vi "Sort 1D Array (U8)__ogtk.vi"(9 "Order":enum16{"ascending", "descending"}(ring), 11 "Array in":u8[](array[numeric])) -> (2 "Sorted Pointers":i32[](array[numeric]), 3 "Sorted Array out":u8[](array[numeric]))   [LabVIEW 2018]
doc: "This polymorphic VI sorts a 1D array of numerics or strings, regardless of the array size. You can specify whether to sort in ascending or descending order."
panel:
  # "Sort 1D Array\n\nThis VI sorts a 1D array of any size in descending or ascending order.\n\nPlease visit http://www.OpenG.org to learn about the\nOpen Source LabVIEW software movement.\n\nNOTICE -- YOU MUST LEAVE THIS NOTICE IN PLACE.  PER THE TERMS OF THE LICENSE BELOW, YOU MAY SUBLICENSE THIS SOFTWARE \nIN ANY WAY THAT DOES NOT CONFLICT WITH THIS LICENSE.\n\n### BSD License (http://www.opensource.org/licenses/bsd-license.php) Begin ###\n \nCopyright (c) 2002, Jim Kring <jim@jimkring.com>\nCopyright (c) 2002, Cal-Bay Systems, Inc. <info@calbay.com>\nCopyright (c) 2005, MKS Instruments, Inc., author: Doug Femec<doug_femec@mksinst.com>, IM dafemec\n\nAll rights reserved.\n\nRedistribution and use in source and binary forms, with or without modification, are permitted provided that the following conditions are met:\n\n    * Redistributions of source code must retain the above copyright notice, this list of conditions and the following disclaimer.\n    * Redistributions in binary form must reproduce the above copyright notice, this list of conditions and the following disclaimer in the \n       documentation and/or other materials provided with the distribution.\n    * Neither the name of SciWare, James Kring, Inc., nor the names of its contributors may be used to endorse or promote products derived \n       from this software without specific prior written permission.\n\nTHIS SOFTWARE IS PROVIDED BY THE COPYRIGHT HOLDERS AND CONTRIBUTORS \"AS IS\" AND ANY EXPRESS OR IMPLIED WARRANTIES, \nINCLUDING, BUT NOT LIMITED TO, THE IMPLIED WARRANTIES OF MERCHANTABILITY AND FITNESS FOR A PARTICULAR PURPOSE ARE \nDISCLAIMED. IN NO EVENT SHALL THE COPYRIGHT OWNER OR CONTRIBUTORS BE LIABLE FOR ANY DIRECT, INDIRECT, INCIDENTAL,\n SPECIAL, EXEMPLARY, OR CONSEQUENTIAL DAMAGES (INCLUDING, BUT NOT LIMITED TO, PROCUREMENT OF SUBSTITUTE GOODS OR \nSERVICES; LOSS OF USE, DATA, OR PROFITS; OR BUSINESS INTERRUPTION) HOWEVER CAUSED AND ON ANY THEORY OF LIABILITY, \nWHETHER IN CONTRACT, STRICT LIABILITY, OR TORT (INCLUDING NEGLIGENCE OR OTHERWISE) ARISING IN ANY WAY OUT OF THE USE \nOF THIS SOFTWARE, EVEN IF ADVISED OF THE POSSIBILITY OF SUCH DAMAGE.\n\n### BSD License End ###"
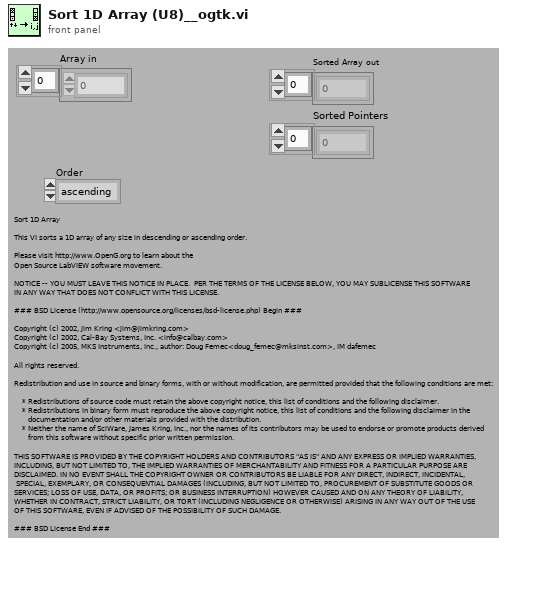
[diagram p1: front panel]
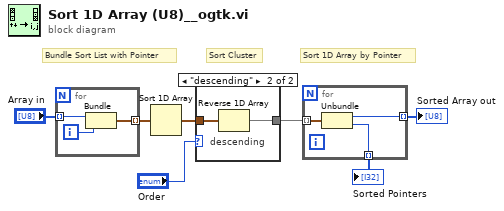
[diagram p0: block diagram]
diagram:
  # "Sort 1D Array by Pointer"
  # "Sort Cluster"
  # "Bundle Sort List with Pointer"
  n1 = for {
    tunnel: "Array in" -> [w10] mode=indexing
    tunnel: [w8] -> w5 mode=indexing
    i -> [w9]
    n2 = Bundle("Numeric"=w10, w9) -> (w8:cluster{"Numeric":u8, i32})  [unwired: 1 in]
  }
  n3 = Sort 1D Array(array=w5) -> (sorted array=w4:cluster{"Numeric":u8, i32}[])
  n4 = case shown="\"descending\"" "Order" {
    tunnel: [w11 w12] -> w6
    tunnel: w4 -> [w11 w13]
    frame "ascending", Default {
    }
    frame "descending" {
      # "descending"
      n5 = Reverse 1D Array(array=w13) -> (reversed array=w12:cluster{"Numeric":u8, i32}[])
    }
  }
  n6 = for {
    tunnel: w6 -> [w16] mode=indexing
    tunnel: [w14] -> w1 mode=indexing
    tunnel: [w15] -> w3 mode=indexing
    n7 = Unbundle(w16) -> ("Numeric"=w14:u8, w15:i32)
  }
  "Sorted Array out" <- w1
  "Sorted Pointers" <- w3
